vi "Set_Ref_Parameters.vi"(8 "error in":errorcluster, 10 "use_increment_halfrate":bool) -> (0 "error out":errorcluster, 2 "index":i32, 3 "FPGA VI Reference Out":T1)   [LabVIEW 2020]
uses:
  RIG-SPECIFIC FILES/FPGA Refs/FPGA Ref.ctl
  Global Variables/FPGAstatus_Reference.vi
  <vilib>/Utility/error.llb/Error Cluster From Error Code.vi
  <vilib>/rvi/errors/niLvFpgaAdjustHostInterfaceError.vi
  <vilib>/rvi/interface/nirviReadWriteControl/nirviReadWriteControl.xnode
  NiFpgaLv.dll
  <vilib>/rvi/interface/Simulation/niFpgaSimulationCallBeginRW.vi
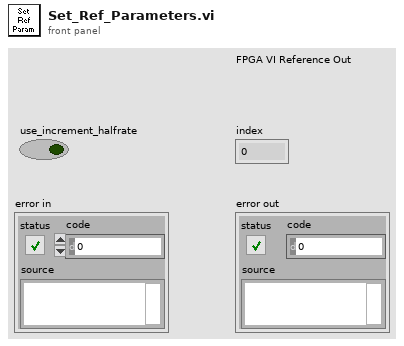
[diagram p1: front panel]
types:
  T1 = typedef "FPGA Ref.ctl" = refnum<k20>
  T2 = typedef "test_fpga_control.ctl" = cluster{"x_offset_host":fxp<+/-,16,8>, "y_offset_host":fxp<+/-,16,8>, "use host offset":bool, "Set_Ref_Centroid":bool, "OldChirpCode":bool, "use array of offsets":bool, "x_offset_host array":fxp<+/-,16,8>[], "y_offset_host array ":fxp<+/-,16,8>[], "use host offset Z":bool, "swap Z":bool, "z_offset_host ":fxp<+/-,16,8>}
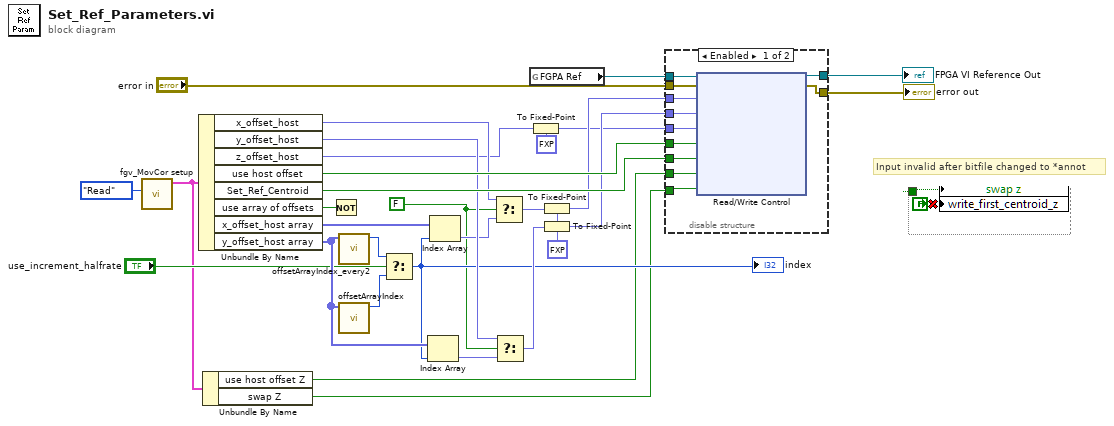
[diagram p0: block diagram]
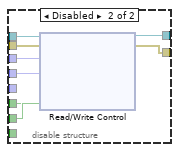
[diagram p2: hidden frame]
diagram:
  w1 = FALSE
  w13 = fxp<+/-,16,8> data[17B] ("x_offset_host")
  # "Input invalid after bitfile changed to *annot"
  n1 = call "fgv_MovCor setup.vi"("Status"=enum16{"Initialize", "Write", "Read"}."Read") -> ("MovCor Cluster"=w7:T2)  [unwired: 9 in, 1 out]
  n2 = Unbundle By Name(w7) -> ("x_offset_host"=w26:fxp<+/-,16,8>, "y_offset_host"=w24:fxp<+/-,16,8>, "z_offset_host"=w4:fxp<+/-,16,8>, "use host offset"=w29:bool, "Set_Ref_Centroid"=w30:bool, "use array of offsets"=w18:bool, "x_offset_host array"=w27:fxp<+/-,16,8>[], "y_offset_host array"=w17:fxp<+/-,16,8>[])
  n3 = Unbundle By Name(w7) -> ("use host offset Z"=w6:bool, "swap Z"=w5:bool)
  n4 = Not(x=w18) -> ()  [unwired: 1 out]
  n5 = call "offsetArrayIndex_every2.vi"("y_offset_host array"=w17) -> ("index"=w16:i32)  [unwired: 10 in]
  n6 = call "offsetArrayIndex.vi"("y_offset_host array"=w17) -> ("index"=w15:i32)  [unwired: 10 in]
  n7 = Select(t=w16, s="use_increment_halfrate", f=w15) -> (s? t:f=w14:i32)
  "index" <- w14
  n8 = Index Array(array=w17, index=w14) -> (element=w19:fxp<+/-,16,8>)
  n9 = Index Array(array=w27, index=w14) -> (element=w20:fxp<+/-,16,8>)
  n10 = Select(t=w26, s=w1, f=w20) -> (s? t:f=w25:fxp<+/-,16,8>)
  n11 = Select(t=w24, s=w1, f=w19) -> (s? t:f=w23:fxp<+/-,16,8>)
  n12 = global read "FPGAstatus_Reference.vi" "FGPA Ref"() -> (w8:T1)
  n13 = To Fixed-Point(fixed-point type=fxp<+/-,16,8> data[17B] ("x_offset_host"), number=w4) -> (fixed-point=w3:fxp<+/-,16,8>)
  n14 = To Fixed-Point(fixed-point type=w13, number=w25) -> (fixed-point=w22:fxp<+/-,16,8>)
  n15 = To Fixed-Point(fixed-point type=w13, number=w23) -> (fixed-point=w21:fxp<+/-,16,8>)
  n16 = disable-structure shown="Enabled" {
    disable-tunnel: w30 -> [w41 w49]
    disable-tunnel: w29 -> [w40 w48]
    disable-tunnel: w22 -> [w39 w47]
    disable-tunnel: w21 -> [w38 w46]
    disable-tunnel: "error in" -> [w37 w45]
    disable-tunnel: [w36 w44] -> w11
    disable-tunnel: [w35 w43] -> w10
    disable-tunnel: w8 -> [w34 w42]
    disable-tunnel: w6 -> [w33 _]
    disable-tunnel: w5 -> [w32 _]
    disable-tunnel: w3 -> [w31 _]
    frame Enabled {
      n17 = xnode "Read/Write Control"("FPGA VI Reference In"=w34, "error in"=w37, "x_offset_host"=w39, "y_offset_host"=w38, "z_offset_host"=w31, "use host offset"=w40, "set_reference"=w41, "use_host_offset_z"=w33, "swap z"=w32) -> ("FPGA VI Reference Out"=w36:T1, "error out"=w35:errorcluster)
    }
    frame Disabled {
      n18 = xnode "Read/Write Control"("FPGA VI Reference In"=w42, "error in"=w45, "x_offset_host"=w47, "y_offset_host"=w46, "use host offset"=w48, "set_reference"=w49) -> ("FPGA VI Reference Out"=w44:T1, "error out"=w43:errorcluster)
    }
  }
  "FPGA VI Reference Out" <- w11
  "error out" <- w10
